vi "Create User Event - Stop.vi"(8 "error in (no error)":errorcluster) -> (0 "error out":errorcluster, 3 "User Event - Stop":refnum<user-event>)   [LabVIEW 2016, in "testData User Event - Stop.lvlib"]
doc: "Create a boolean user event that will be used to stop the event loop from the message handling loop."
uses:
  testData User Event - Stop.lvlib
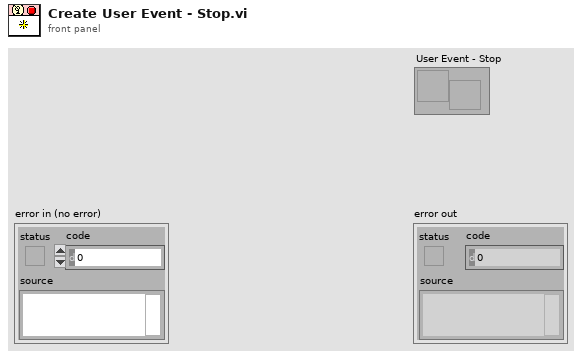
[diagram p1: front panel]
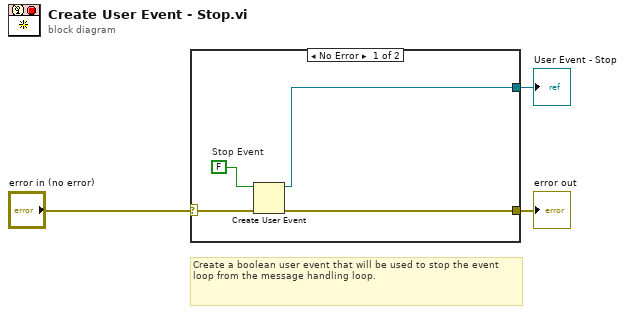
[diagram p0: block diagram]
diagram:
  # "Create a boolean user event that will be used to stop the event loop from the message handling loop."
  n1 = case shown="No Error" "error in (no error)" {
    selector: "error in (no error)" -> [w4 w8]
    tunnel: [w7 _] -> w3
    tunnel: [w5 w8] -> w2
    frame No Error {
      w6 = FALSE  # Stop Event
      n2 = Create User Event(user event datatype=w6, error in=w4) -> (user event=w7:refnum<user-event>, error out=w5:errorcluster)
    }
    frame Error {
    }
  }
  "User Event - Stop" <- w3
  "error out" <- w2
